vi "信号发生器2.0【波形图】.vi"() -> ()   [LabVIEW 2022 SP3]
uses:
  <vilib>/Analysis/baseanly.llb/Mean (DBL).vi
  <vilib>/measure/NI_MABase.lvlib
  <vilib>/measure/NI_MAPro.lvlib
  <vilib>/Analysis/NI_AALBase.lvlib
panel:
  out "开始指示灯":bool
  in  "信号发生器开关":bool
  out "波形信息":string
  out "波形编号":i64
  out "程序中止指示灯":bool
  out "中间类型":string
  out "中间保存数组":dbl[](array[numeric])
  in  "保存":bool
  out "波形图":dbl[](graph)
  out "算数平均值":dbl
  out "最小值":dbl
  out "最大值":dbl
  in  "停止":bool
  in  "保存路径":path
  in  "自定义公式":string
  in  "采样数":i64(knob) scale=1.0..1000.0
  in  "采样率":i64(knob) scale=150.0..1500.0
  in  "偏移量":i64(knob) scale=-20.0..20.0
  in  "标准差（高斯白噪声）":i64(knob) scale=0.0..10.0
  in  "幅度":i64(knob) scale=0.0..30.0
  in  "频率":i64(knob) scale=0.0..50.0
  in  "波形类型":u16(ring) items=["三角波", "正弦波", "自定义波形", "方波", "锯齿波"]
  # "信号发生器"
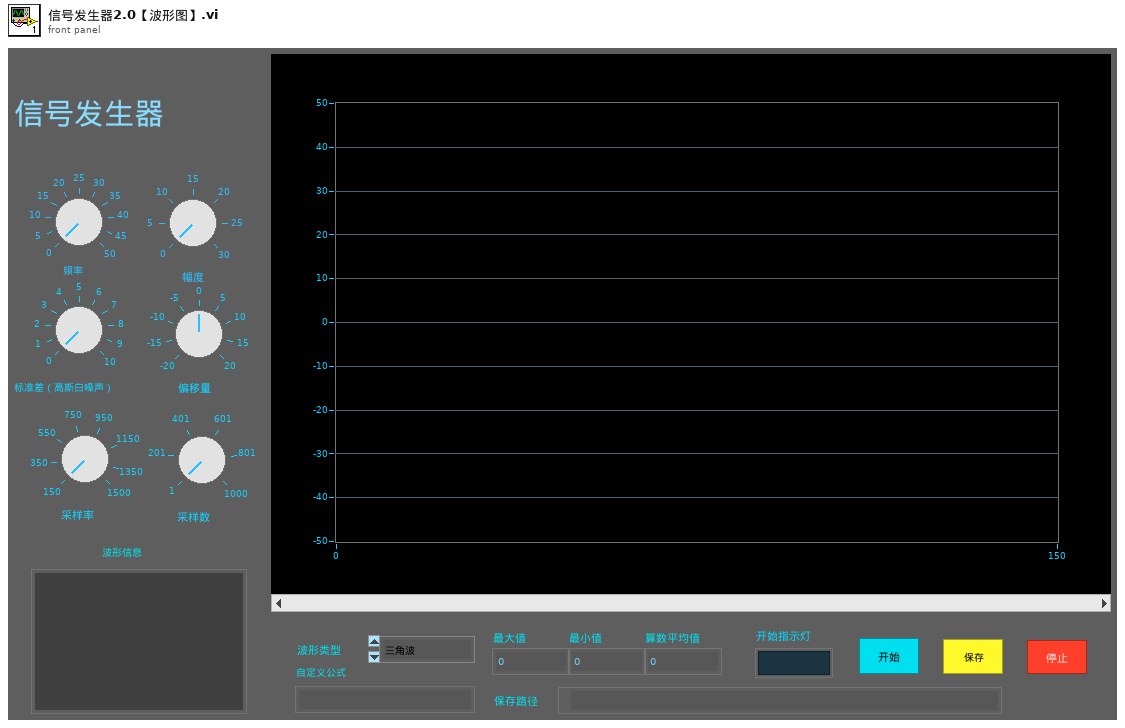
[diagram p1: front panel]
types:
  T1 = enum16{"open", "replace", "create", "open or create", "replace or create", "replace or create with confirmation"}
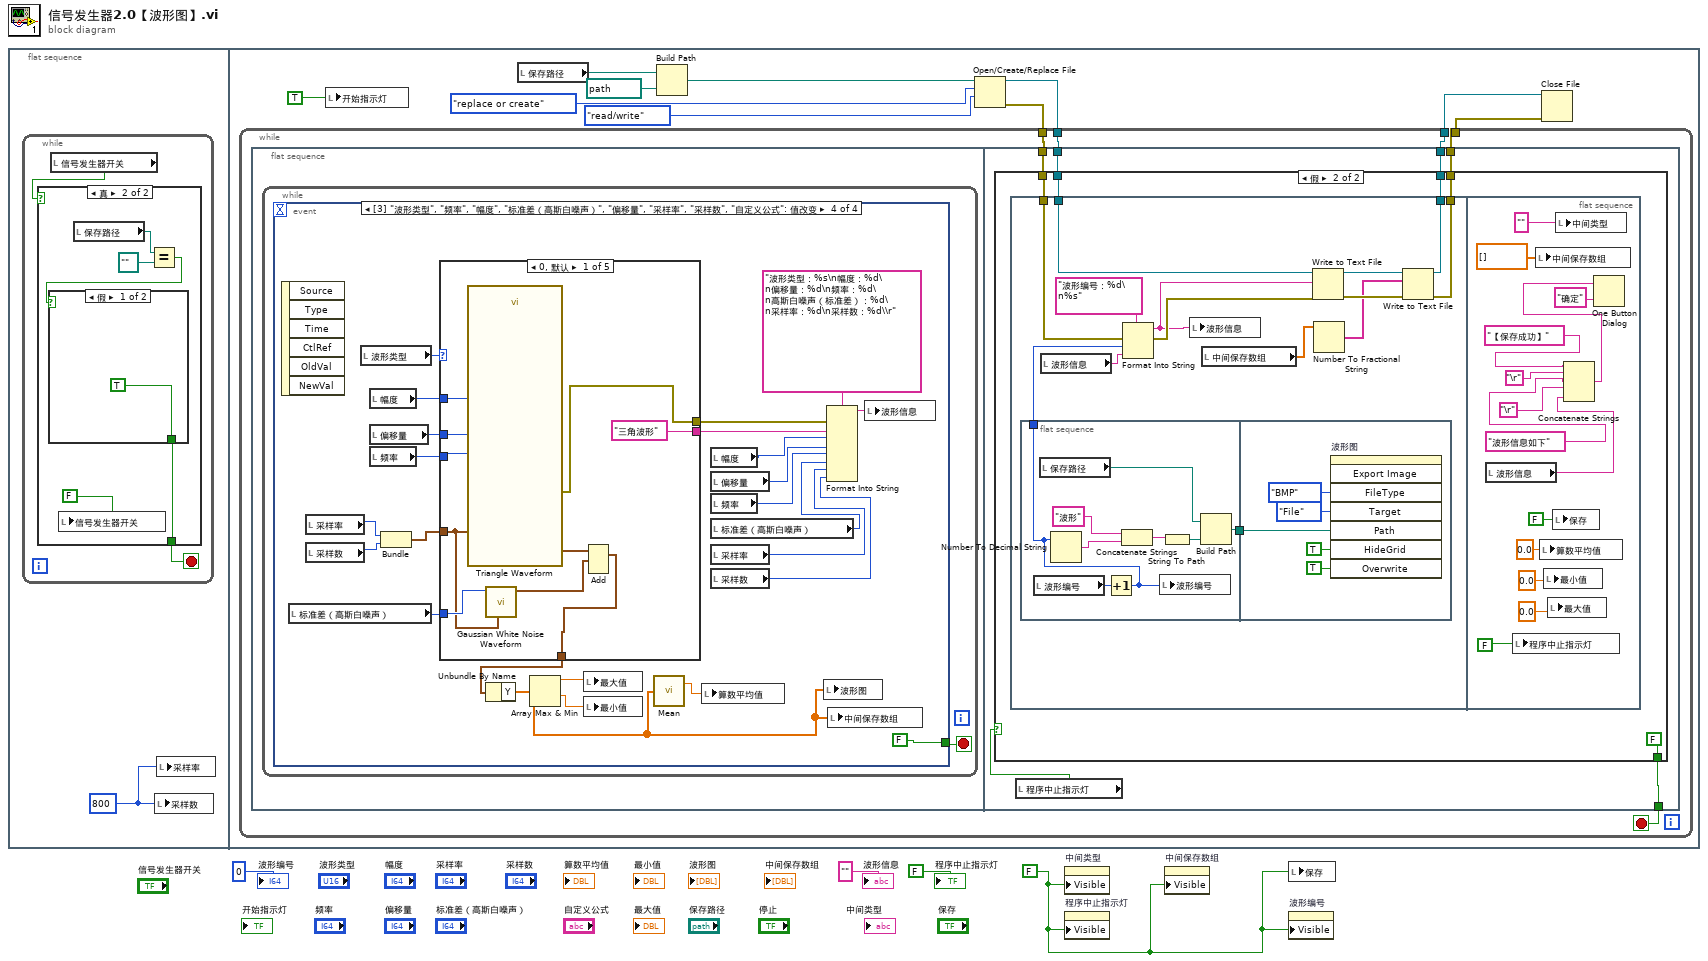
[diagram p0: block diagram]
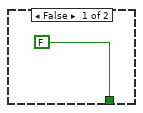
[diagram p2: hidden frame]
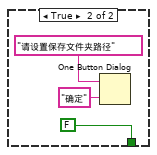
[diagram p3: hidden frame]
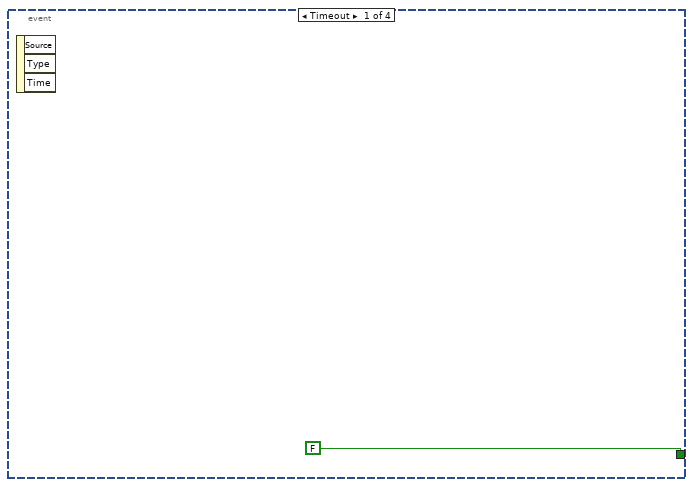
[diagram p4: hidden frame]
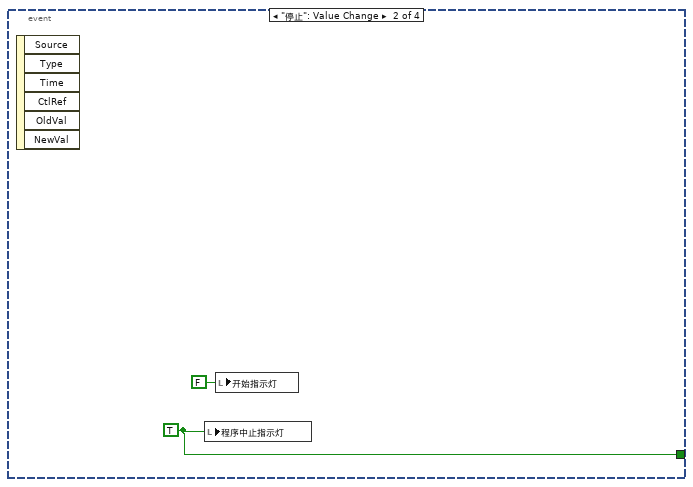
[diagram p5: hidden frame]
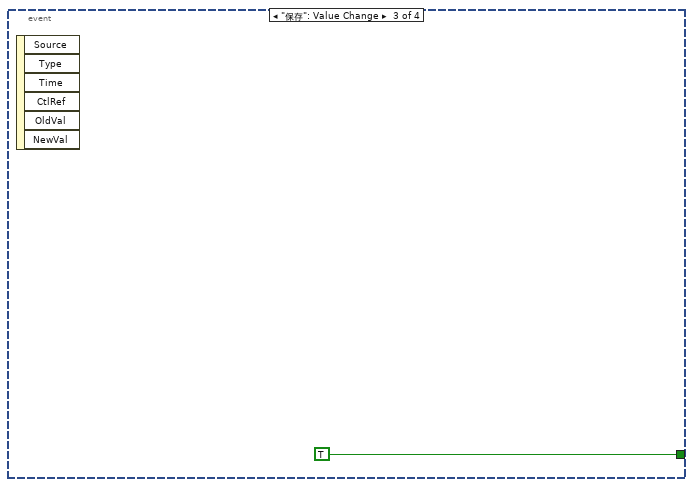
[diagram p6: hidden frame]
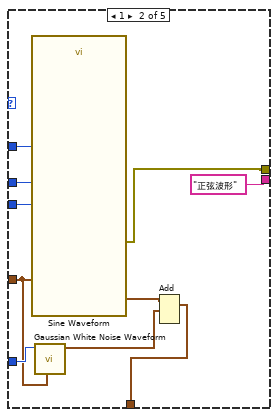
[diagram p7: hidden frame]
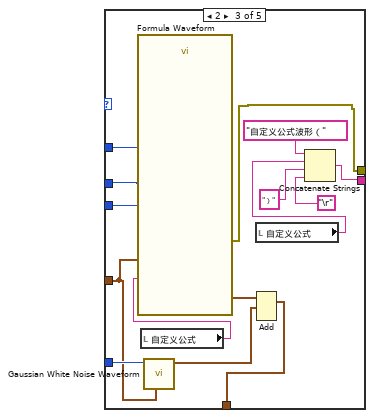
[diagram p8: hidden frame]
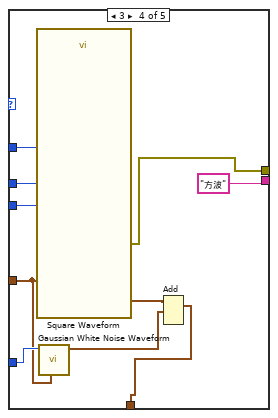
[diagram p9: hidden frame]
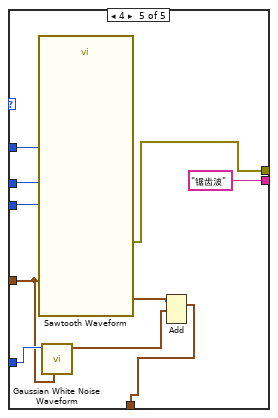
[diagram p10: hidden frame]
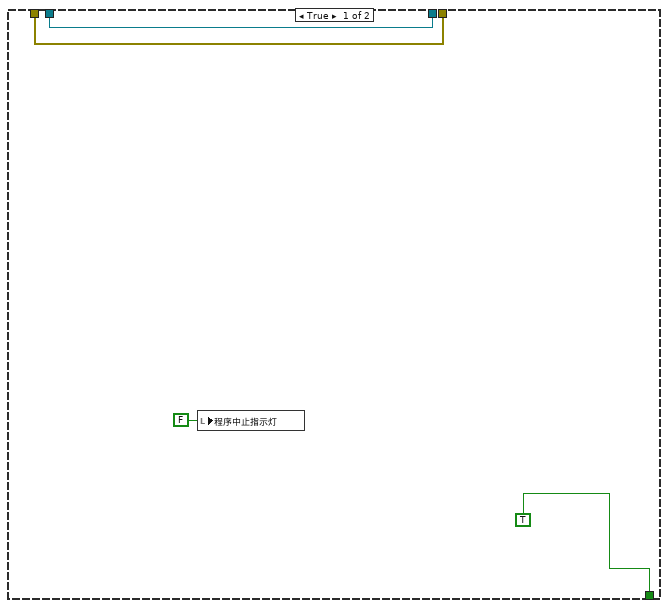
[diagram p11: hidden frame]
diagram:
  w2 = FALSE ("可见")
  n1 = flat-sequence {
    frame #0 {
      w5 = i64 800 ("采样数")
      n2 = while {
        stop <- w6 stop-if-true
        n3 = local read "信号发生器开关"() -> (w7:bool)
        n4 = case shown="真" w7 {
          tunnel: [FALSE w10] -> w6
          frame False {
          }
          frame True {
            n5 = local write "信号发生器开关"(FALSE) -> ()
            n6 = local read "保存路径"() -> (w13:path)
            n7 = Equal?(x=w13, y=path "") -> (x = y?=w11:bool)
            n8 = case shown="假" w11 {
              tunnel: [TRUE FALSE] -> w10
              frame False {
              }
              frame True {
                n9 = One Button Dialog(message="请设置保存文件夹路径" ("消息"), button name ("OK")="确定" ("按钮名称（“确定”）")) -> ()  [unwired: 1 out]
              }
            }
          }
        }
      }
      n10 = local write "采样数"(w5) -> ()
      n11 = local write "采样率"(w5) -> ()
    }
    frame #1 {
      n12 = local write "开始指示灯"(TRUE) -> ()
      n13 = local read "保存路径"() -> (w19:path)
      n14 = Build Path(base path=w19, name or relative path=path "记录.txt") -> (appended path=w26:path)
      n15 = Open/Create/Replace File(file path (use dialog)=w26, operation (0:open)=T1."replace or create" ("操作(0:open)"), access (0:read/write)=enum16{"read/write", "read-only", "write-only"}."read/write" ("权限(0:read/write)")) -> (refnum out=w22:refnum<file>, error out=w23:errorcluster)  [unwired: 3 in, 1 out]
      n16 = while {
        tunnel: w23 -> [w29]
        tunnel: w22 -> [w28]
        tunnel: [w32] -> w21
        tunnel: [w31] -> w20
        stop <- w30 stop-if-true
        n17 = flat-sequence {
          tunnel: w28 -> [w122]
          tunnel: [w121] -> w32
          tunnel: [w120] -> w31
          tunnel: [w117] -> w30
          tunnel: w29 -> [w118]
          frame #0 {
            n18 = while {
              stop <- w33 stop-if-true
              n19 = event shown="[3] \"波形类型\", \"频率\", \"幅度\", \"标准差（高斯白噪声）\", \"偏移量\", \"采样率\", \"采样数\", \"自定义公式\": 值改变" {
                selector: _ -> [_ _ _ _]
                dyn-events: _ -> [_ _ _ _]
                timeout: _ -> [_ _ _ _]
                tunnel: [FALSE w36 TRUE FALSE] -> w33
                event Timeout {
                  n20 = event-data() -> ()  [unwired: 1 in, 3 out]
                }
                event "停止": Value Change {
                  w36 = TRUE ("停止？(T)")
                  n21 = event-data() -> ()  [unwired: 1 in, 6 out]
                  n22 = local write "程序中止指示灯"(w36) -> ()
                  n23 = local write "开始指示灯"(FALSE ("开始指示灯")) -> ()
                }
                event "保存": Value Change {
                  n24 = event-data() -> ()  [unwired: 1 in, 6 out]
                }
                event "波形类型", "频率", "幅度", "标准差（高斯白噪声）", "偏移量", "采样率", "采样数", "自定义公式": Value Change {
                  n25 = event-data() -> ()  [unwired: 1 in, 6 out]
                  n26 = local read "标准差（高斯白噪声）"() -> (w60:i64)
                  n27 = local read "采样率"() -> (w56:i64)
                  n28 = local read "采样数"() -> (w55:i64)
                  n29 = local read "波形类型"() -> (w61:u16)
                  n30 = local read "幅度"() -> (w57:i64)
                  n31 = local read "偏移量"() -> (w58:i64)
                  n32 = local read "频率"() -> (w59:i64)
                  n33 = Bundle("采样率"=w56, "采样数"=w55) -> (w54:cluster{"采样率":i64, "采样数":i64})  [unwired: 1 in]
                  n34 = case shown="0, 默认" w61 {
                    tunnel: w60 -> [w68 w78 w91 w100 w111]
                    tunnel: w59 -> [w69 w79 w96 w103 w112]
                    tunnel: w58 -> [w70 w80 w95 w102 w113]
                    tunnel: w57 -> [w71 w81 w94 w101 w114]
                    tunnel: w54 -> [w67 w77 w90 w99 w109]
                    tunnel: [w64 w74 w84 w104 w110] -> w49
                    tunnel: ["三角波形" "正弦波形" w83 "方波" "锯齿波"] -> w39
                    tunnel: [w62 w72 w82 w97 w107] -> w38
                    frame 0, Default {
                      n35 = call <vilib>:"Triangle Waveform.vi"("offset"=w70, "sampling info"=w67, "amplitude"=w71, "frequency"=w69) -> ("error out"=w62:errorcluster, "signal out"=w66:waveform(dbl))  [unwired: 6 in]
                      n36 = call <vilib>:"Gaussian White Noise Waveform.vi"("sampling info"=w67, "standard deviation"=w68) -> ("signal out"=w65:waveform(dbl))  [unwired: 8 in, 1 out]
                      n37 = Add(1:w65, 2:w66) -> (0:w64:waveform(dbl))  [unwired: 1 in, 1 out]
                    }
                    frame 1 {
                      n38 = call <vilib>:"Sine Waveform.vi"("offset"=w80, "sampling info"=w77, "amplitude"=w81, "frequency"=w79) -> ("error out"=w72:errorcluster, "signal out"=w76:waveform(dbl))  [unwired: 6 in]
                      n39 = call <vilib>:"Gaussian White Noise Waveform.vi"("sampling info"=w77, "standard deviation"=w78) -> ("signal out"=w75:waveform(dbl))  [unwired: 8 in, 1 out]
                      n40 = Add(1:w75, 2:w76) -> (0:w74:waveform(dbl))  [unwired: 1 in, 1 out]
                    }
                    frame 2 {
                      n41 = local read "自定义公式"() -> (w93:string)
                      n42 = call <vilib>:"Formula Waveform.vi"("offset"=w95, "sampling info"=w90, "formula"=w93, "amplitude"=w94, "frequency"=w96) -> ("error out"=w82:errorcluster, "signal out"=w92:waveform(dbl))  [unwired: 5 in]
                      n43 = call <vilib>:"Gaussian White Noise Waveform.vi"("sampling info"=w90, "standard deviation"=w91) -> ("signal out"=w89:waveform(dbl))  [unwired: 8 in, 1 out]
                      n44 = Add(1:w89, 2:w92) -> (0:w84:waveform(dbl))  [unwired: 1 in, 1 out]
                      n45 = local read "自定义公式"() -> (w87:string)
                      n46 = Concatenate Strings("自定义公式波形（", w87, "）" ("字符串"), "\r") -> (w83:string)
                    }
                    frame 3 {
                      n47 = call <vilib>:"Square Waveform.vi"("offset"=w102, "sampling info"=w99, "amplitude"=w101, "frequency"=w103) -> ("error out"=w97:errorcluster, "signal out"=w106:waveform(dbl))  [unwired: 6 in]
                      n48 = call <vilib>:"Gaussian White Noise Waveform.vi"("sampling info"=w99, "standard deviation"=w100) -> ("signal out"=w105:waveform(dbl))  [unwired: 8 in, 1 out]
                      n49 = Add(1:w105, 2:w106) -> (0:w104:waveform(dbl))  [unwired: 1 in, 1 out]
                    }
                    frame 4 {
                      n50 = call <vilib>:"Sawtooth Waveform.vi"("offset"=w113, "sampling info"=w109, "amplitude"=w114, "frequency"=w112) -> ("error out"=w107:errorcluster, "signal out"=w116:waveform(dbl))  [unwired: 6 in]
                      n51 = call <vilib>:"Gaussian White Noise Waveform.vi"("sampling info"=w109, "standard deviation"=w111) -> ("signal out"=w115:waveform(dbl))  [unwired: 8 in, 1 out]
                      n52 = Add(1:w115, 2:w116) -> (0:w110:waveform(dbl))  [unwired: 1 in, 1 out]
                    }
                  }
                  n53 = Unbundle By Name(w49) -> ("Y"=w50:dbl[])
                  n54 = Array Max & Min(array=w50) -> (max value=w51:dbl, min value=w52:dbl)  [unwired: 2 out]
                  n55 = local write "最大值"(w51) -> ()
                  n56 = local write "最小值"(w52) -> ()
                  n57 = call-poly <vilib>:"Mean.vi"("X"=w50) -> ("mean"=w53:dbl)  [unwired: 1 out]
                  n58 = local write "算数平均值"(w53) -> ()
                  n59 = local read "幅度"() -> (w42:i64)
                  n60 = local read "偏移量"() -> (w43:i64)
                  n61 = local read "频率"() -> (w44:i64)
                  n62 = local read "标准差（高斯白噪声）"() -> (w45:i64)
                  n63 = local read "采样率"() -> (w46:i64)
                  n64 = local read "采样数"() -> (w47:i64)
                  n65 = local write "波形图"(w50) -> ()
                  n66 = Format Into String(format string="波形类型：%s\n幅度：%d\n偏移量：%d\n频率：%d\n高斯白噪声（标准差）：%d\n采样率：%d\n采样数：%d\\r", error in=w38, w39, w42, w43, w44, w45, w46, w47) -> (resulting string=w40:string)  [unwired: 1 in, 1 out]
                  n67 = local write "中间保存数组"(w50) -> ()
                  n68 = local write "波形信息"(w40) -> ()
                }
              }
            }
          }
          frame #1 {
            n69 = local read "程序中止指示灯"() -> (w119:bool)
            n70 = case shown="假" w119 {
              tunnel: w122 -> [w126 w131]
              tunnel: w118 -> [w125 w130]
              tunnel: [w125 w129] -> w121
              tunnel: [w126 w128] -> w120
              tunnel: [TRUE FALSE] -> w117
              frame True {
                n71 = local write "程序中止指示灯"(FALSE ("程序中止指示灯")) -> ()
              }
              frame False {
                n72 = flat-sequence {
                  tunnel: w131 -> [w145]
                  tunnel: w130 -> [w136]
                  tunnel: [w141] -> w129
                  tunnel: [w140] -> w128
                  frame #0 {
                    n73 = flat-sequence {
                      tunnel: [w151] -> w138
                      tunnel: [w146] -> w135
                      tunnel: w138 -> [w154]
                      frame #0 {
                        n74 = local read "波形编号"() -> (w153:i64)
                        n75 = local read "保存路径"() -> (w152:path)
                        n76 = Increment(x=w153) -> (x+1=w146:i64)
                        n77 = Number To Decimal String(number=w146) -> (decimal integer string=w149:string)  [unwired: 1 in]
                        n78 = Concatenate Strings("波形" ("连接的字符串"), w149) -> (w148:string)
                        n79 = local write "波形编号"(w146) -> ()
                        n80 = String To Path(string=w148) -> (path=w150:path)
                        n81 = Build Path(base path=w152, name or relative path=w150) -> (appended path=w151:path)
                      }
                      frame #1 {
                        n82 = invoke on="波形图" class="WFGraph (严格)" method="Export Image"("FileType"=enum32{"BMP", "EPS", "EMF", "PICT"}."BMP" ("文件类型"), "Target"=enum32{"File", "Clipboard"}."File" ("目标"), "Path"=w154, "HideGrid"=TRUE ("隐藏网格"), "Overwrite"=TRUE ("始终覆盖")) -> ()  [unwired: 3 in, 8 out]
                      }
                    }
                    n83 = local read "波形信息"() -> (w134:string)
                    n84 = Format Into String(format string="波形编号：%d\n%s", error in=w136, w135, w134) -> (resulting string=w132:string, error out=w133:errorcluster)  [unwired: 1 in]
                    n85 = local write "波形信息"(w132) -> ()
                    n86 = local read "中间保存数组"() -> (w139:dbl[])
                    n87 = Write to Text File(file (use dialog)=w145, text=w132, error in=w133) -> (refnum out=w144:refnum<file>, error out=w143:errorcluster)  [unwired: 1 in, 1 out]
                    n88 = Number To Fractional String(number=w139) -> (F-format string=w142:string[])  [unwired: 3 in]
                    n89 = Write to Text File(file (use dialog)=w144, text=w142, error in=w143) -> (refnum out=w140:refnum<file>, error out=w141:errorcluster)  [unwired: 1 in, 1 out]
                  }
                  frame #1 {
                    n90 = local read "波形信息"() -> (w159:string)
                    n91 = local write "程序中止指示灯"(FALSE) -> ()
                    n92 = local write "中间保存数组"(dbl[] [] ("中间保存数组")) -> ()
                    n93 = local write "算数平均值"(0.0 ("算数平均")) -> ()
                    n94 = local write "最小值"(0.0 ("最小值")) -> ()
                    n95 = local write "最大值"(0.0 ("最大值")) -> ()
                    n96 = local write "保存"(FALSE ("保存")) -> ()
                    n97 = local write "中间类型"("" ("中间类型字符串")) -> ()
                    n98 = Concatenate Strings("【保存成功】" ("消息"), "\r", "波形信息如下", "\r", w159) -> (w164:string)
                    n99 = One Button Dialog(message=w164, button name ("OK")="确定" ("按钮名称（“确定”）")) -> ()  [unwired: 1 out]
                  }
                }
              }
            }
          }
        }
      }
      n100 = Close File(refnum=w20, error in=w21) -> ()  [unwired: 2 out]
    }
  }
  n101 = property on="中间类型" class="Str"("Visible"=w2) -> ()  [unwired: 2 in, 2 out]
  n102 = property on="程序中止指示灯" class="Bool (严格)"("Visible"=w2) -> ()  [unwired: 2 in, 2 out]
  n103 = property on="中间保存数组" class="Arr (严格)"("Visible"=w2) -> ()  [unwired: 2 in, 2 out]
  n104 = local write "保存"(w2) -> ()
  n105 = property on="波形编号" class="DigNum (严格)"("Visible"=w2) -> ()  [unwired: 2 in, 2 out]
  "程序中止指示灯" <- FALSE
  "波形编号" <- i64 0 ("波形编号")
  "波形信息" <- "" ("波形信息")
